vi "Mem_Str.vi"(8 "error in (no error)":errorcluster, 11 "dataInfo":T1) -> (0 "error out":errorcluster, 2 "response":string)   [LabVIEW 2019, in "Memory Data Access.lvlib"]
uses:
  Memory Data Access.lvlib
  Typedef/memoryDataBlock.ctl
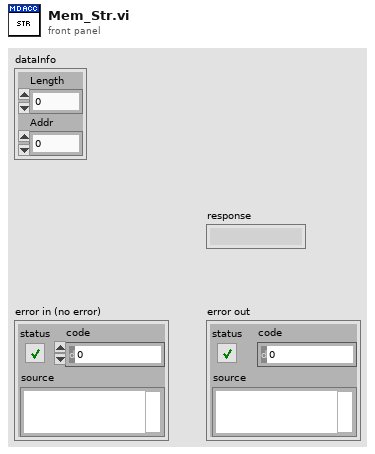
[diagram p1: front panel]
types:
  T1 = typedef "Memory Data Access.lvlib/memoryDataBlock.ctl" = cluster{"Length":u32, "Addr":u64}
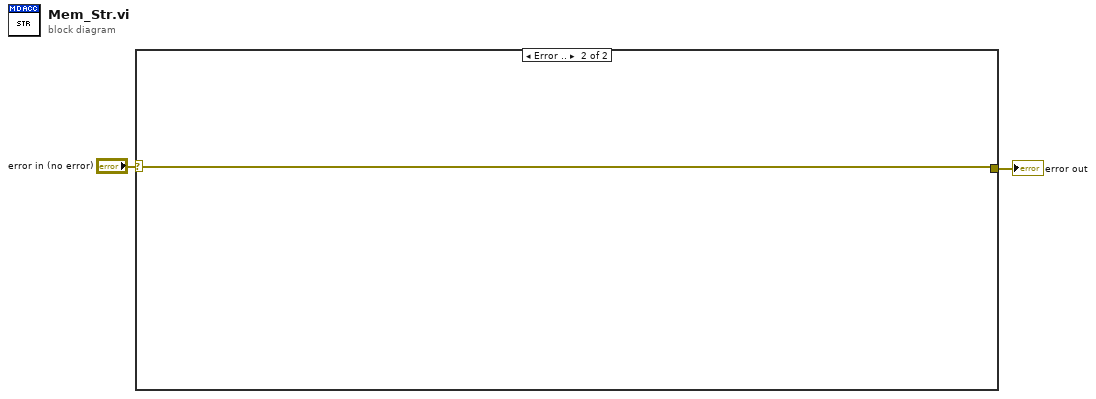
[diagram p0: block diagram]
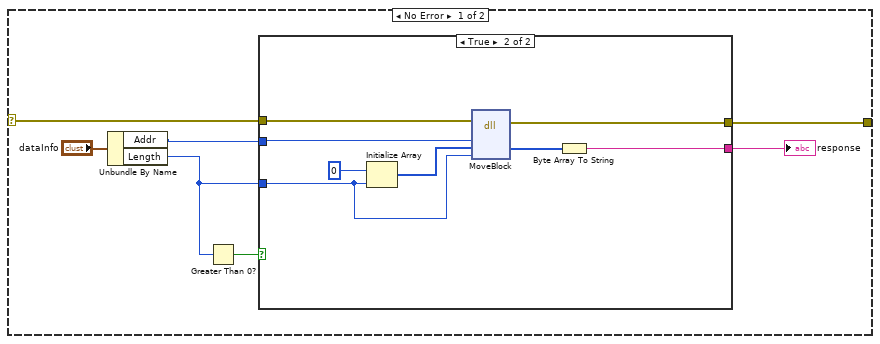
[diagram p2: hidden frame]
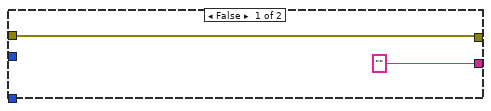
[diagram p3: hidden frame]
diagram:
  n1 = case shown="Error .." "error in (no error)" {
    selector: "error in (no error)" -> [w9 w20]
    tunnel: [w8 w20] -> w1
    frame No Error {
      n2 = Unbundle By Name("dataInfo") -> ("Addr"=w4:u64, "Length"=w3:u32)
      n3 = Greater Than 0?(x=w3) -> (x > 0?=w7:bool)
      n4 = case shown="True" w7 {
        tunnel: w9 -> [w11 w19]
        tunnel: [w11 w18] -> w8
        tunnel: w4 -> [_ w16]
        tunnel: w3 -> [_ w15]
        tunnel: ["" ("string") w12] -> w6
        frame False {
        }
        frame True {
          n5 = Initialize Array(u8 0, w15) -> (w17:u8[])
          n6 = dll-call lib="LabVIEW" fn="MoveBlock"(error in=w19, "Address"=w16, "Destination"=w17, "Size"=w15) -> (error out=w18:errorcluster, "Destination"=w13:u8[])  [unwired: 5 in, 1 out]
          n7 = Byte Array To String(unsigned byte array=w13) -> (string=w12:string)
        }
      }
      "response" <- w6
    }
    frame Error {
    }
  }
  "error out" <- w1
